vi "GetActHFLockInPhase.vi"(5 "error in":T1) -> (14 "Phase":sgl format="%#_g deg", 19 "error out":T1)   [LabVIEW 2016]
doc: "Returns the actual value of the high frequency lock-in phase in degrees."
uses:
  Controls/Error_Out.ctl
  Files_ASC500/DLL/ASC500_RemoteControlV27.dll
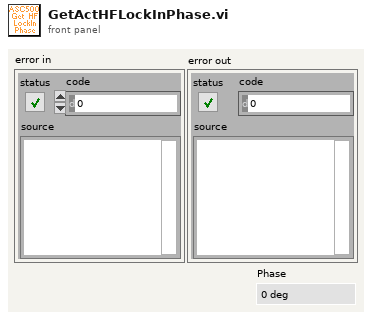
[diagram p1: front panel]
types:
  T1 = typedef "Error_Out.ctl" = errorcluster
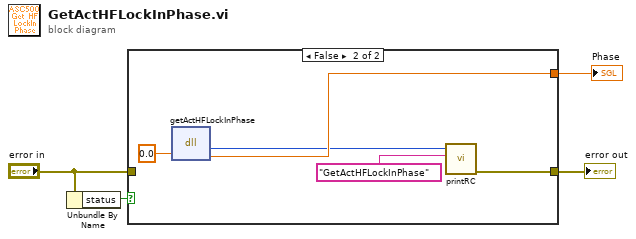
[diagram p0: block diagram]
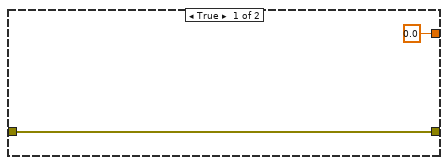
[diagram p2: hidden frame]
diagram:
  n1 = Unbundle By Name("error in") -> ("status"=w4:bool)
  n2 = case shown="False" w4 {
    tunnel: [sgl 0.0 ("Phase") w10] -> w3
    tunnel: "error in" -> [w5 _]
    tunnel: [w5 w8] -> w1
    frame True {
    }
    frame False {
      n3 = dll-call lib="G:/SCMOperations/Share/ELE/Produkt Information/ASC500/04 Remote Control/02 development versions/2018Nov06/Files_ASC500/DLL/ASC500_RemoteControlV27.dll" fn="getActHFLockInPhase"("Phase"=sgl 0.0 ("Amplitude")) -> ("return type"=w9:i32, "Phase"=w10:sgl)  [unwired: 3 in, 2 out]
      n4 = call "printRC.vi"("additional information"="GetActHFLockInPhase", "RC"=w9) -> ("error out"=w8:T1)  [unwired: 9 in]
    }
  }
  "error out" <- w1
  "Phase" <- w3
